vi "Write.vi"(8 "error in (no error)":errorcluster, 10 "command":string, 11 "HAL.TCP in":refnum<class "HAL.TCP.lvclass">) -> (0 "error out":errorcluster, 3 "HAL.TCP out":refnum<class "HAL.TCP.lvclass">)   [LabVIEW 2019, in "Instrument.lvlib" / "HAL.TCP.lvclass"]
doc: "Override to <b>open</b> a connection to your instrument."
uses:
  HAL.TCP.lvclass
  HAL.TCP.lvclass/HAL.TCP.ctl
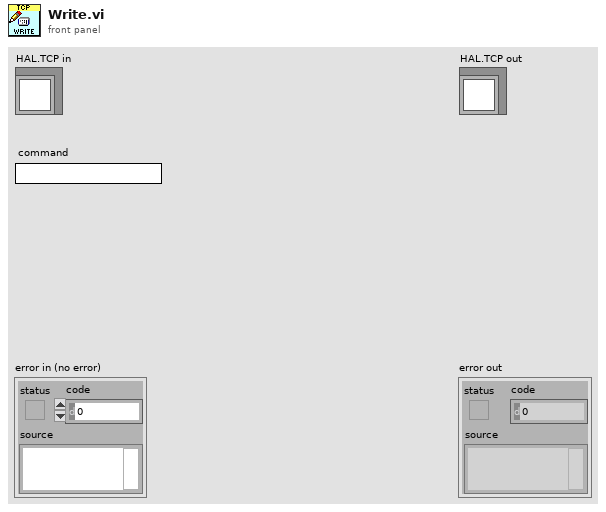
[diagram p1: front panel]
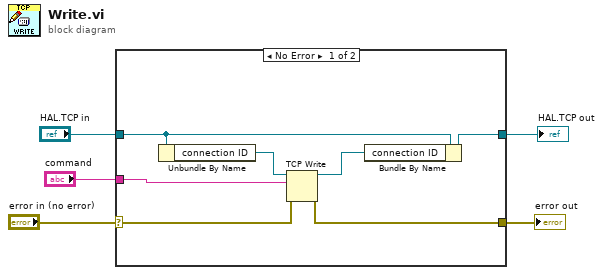
[diagram p0: block diagram]
diagram:
  n1 = case shown="No Error" "error in (no error)" {
    selector: "error in (no error)" -> [w7 w14]
    tunnel: "HAL.TCP in" -> [w12 w13]
    tunnel: [w6 w14] -> w2
    tunnel: [w11 w13] -> w3
    tunnel: "command" -> [w8 _]
    frame No Error {
      n2 = Unbundle By Name(w12) -> ("connection ID"=w10:refnum<k5>)
      n3 = TCP Write(connection ID=w10, data in=w8, error in (no error)=w7) -> (connection ID out=w9:refnum<k5>, error out=w6:errorcluster)  [unwired: 1 in, 1 out]
      n4 = Bundle By Name(cluster=w12, "connection ID"=w9) -> (w11:refnum<class "HAL.TCP.lvclass">)
    }
    frame Error {
    }
  }
  "error out" <- w2
  "HAL.TCP out" <- w3
